vi "Write sampling InfoV2.vi"(8 "error in (no error)":errorcluster, 10 "sampling Info":cluster{"Fs":dbl}={"Fs"=100.0} {"Fs" format="%.2p"}, 11 "ChirpV2 in":refnum<class "ChirpV2.lvclass">) -> (0 "error out":errorcluster, 3 "ChirpV2 out":refnum<class "ChirpV2.lvclass">)   [LabVIEW 2014, in "ChirpV2.lvclass"]
uses:
  ChirpV2.lvclass
  ChirpV2.lvclass/ChirpV2.ctl
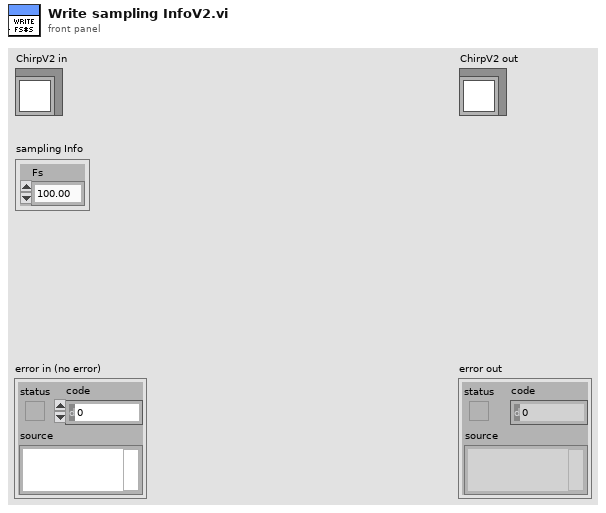
[diagram p1: front panel]
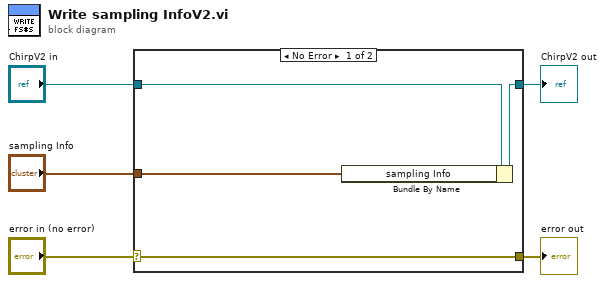
[diagram p0: block diagram]
diagram:
  n1 = case shown="No Error" "error in (no error)" {
    selector: "error in (no error)" -> [w9 w10]
    tunnel: [w9 w10] -> w4
    tunnel: [w7 w11] -> w2
    tunnel: "ChirpV2 in" -> [w8 w11]
    tunnel: "sampling Info" -> [w6 _]
    frame No Error {
      n2 = Bundle By Name(cluster=w8, "sampling Info"=w6) -> (w7:refnum<class "ChirpV2.lvclass">)
    }
    frame Error {
    }
  }
  "error out" <- w4
  "ChirpV2 out" <- w2
